vi "AssertsSubpanelExecStateIdleorRun.vi"(0 "VI Reference In":refnum<vi>, 1 "Label (VI Title)":string="Default", 11 "error in":errorcluster) -> (4 "VI Reference Out":refnum<vi>, 15 "error out":errorcluster)   [LabVIEW 2016, in "DronaTest.lvlib"]
uses:
  APIs/Stimulus/ControlValue/ValueSignalByPathString.vi
  APIs/Stimulus/ControlValue/ValueSignalLatchBooleanString.vi
  APIs/Assert/AssertSubpanel/AssertSubpanelVIExecIdle.vi
  <vilib>/addons/_JKI Toolkits/Caraya/classes/Assert/Assert Not Error.vi
  APIs/Assert/AssertSubpanel/AssertSubpanelVIExecRunning.vi
  APIs/Assert/AssertSubpanel/AssertSubpanelVIExecNotBad.vi
  DronaTest.lvlib
  <vilib>/addons/_JKI Toolkits/Caraya/classes/Test/Test.lvclass
  Drona.lvlib
  <vilib>/addons/_JKI Toolkits/Caraya/classes/Assert/Assert.lvclass
  APIs/Stimulus/ControlValue/ControlValue.lvlib
  APIs/Assert/AssertSubpanel/AssertSubpanel.lvlib
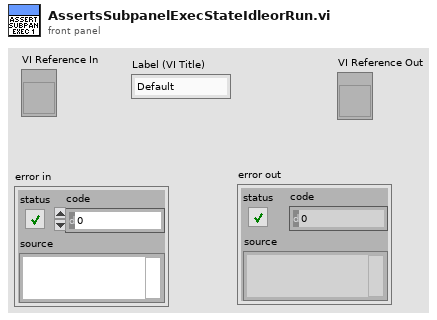
[diagram p1: front panel]
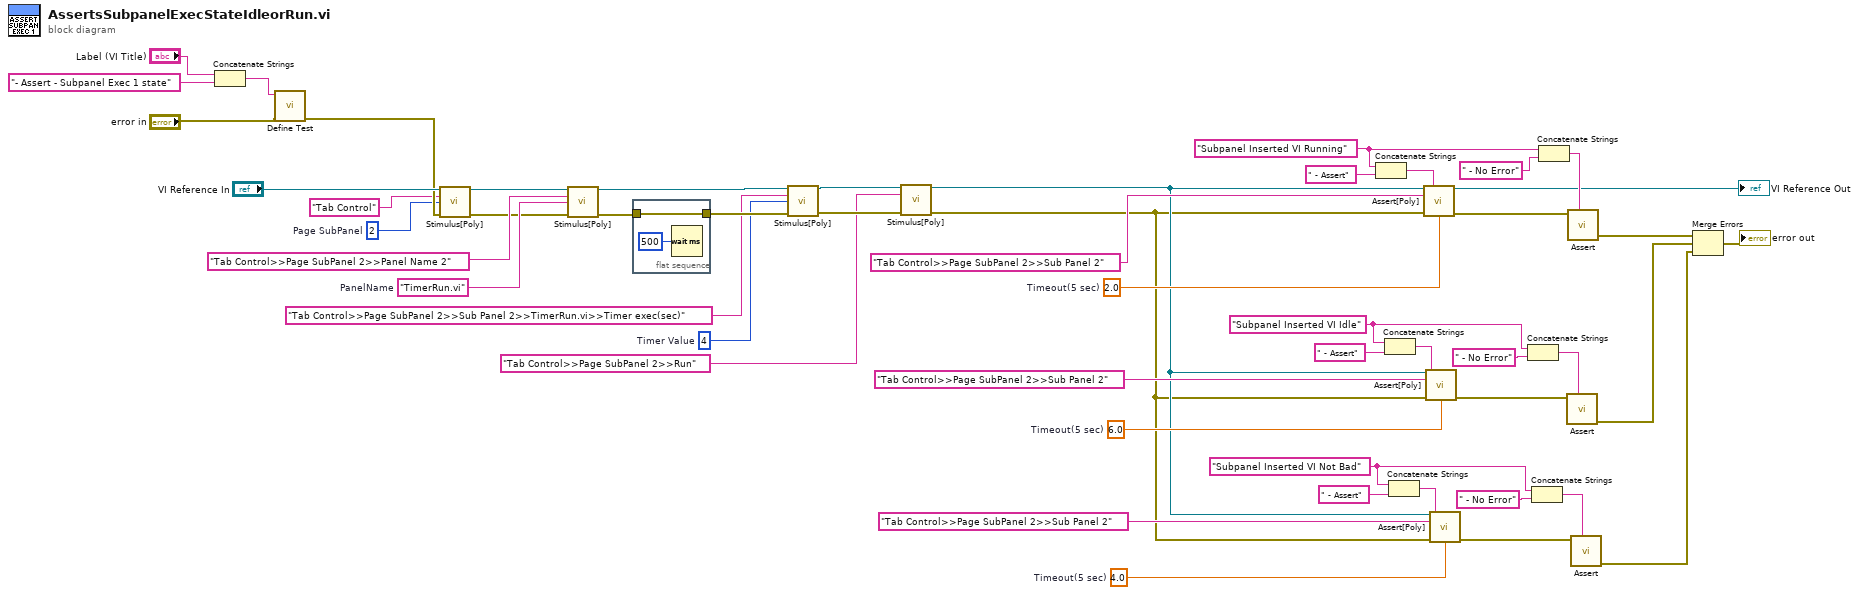
[diagram p0: block diagram]
diagram:
  w1 = 4.0  # Timeout(5 sec)
  w8 = "Subpanel Inserted VI Not Bad" ("Label")
  w16 = 4  # Timer Value
  w20 = 2  # Page SubPanel
  w26 = "TimerRun.vi"  # PanelName
  w36 = "Subpanel Inserted VI Idle" ("Label")
  w39 = "Subpanel Inserted VI Running" ("Label")
  w33 = 6.0  # Timeout(5 sec)
  w29 = 2.0  # Timeout(5 sec)
  n1 = Concatenate Strings("Label (VI Title)", "- Assert - Subpanel Exec 1 state" ("string")) -> (w46:string)
  n2 = call <vilib>:"Define Test.vi"("error in (no error)"="error in", "Label (VI Title)"=w46) -> ("error out"=w22:errorcluster)  [unwired: 9 in]
  n3 = call-poly "Stimulus[Poly].vi"("VI Reference In"="VI Reference In", "Control Path"="Tab Control", "Value (Signaling)"=w20, "error in"=w22) -> ("VI Reference Out"=w23:refnum<vi>, "error out"=w19:errorcluster)  [unwired: 10 in]
  n4 = call-poly "Stimulus[Poly].vi"("VI Reference In"=w23, "Control Path"="Tab Control>>Page SubPanel 2>>Panel Name 2", "Value (Signaling)"=w26, "error in"=w19) -> ("VI Reference Out"=w12:refnum<vi>, "error out"=w25:errorcluster)  [unwired: 10 in]
  n5 = flat-sequence {
    tunnel: w25 -> [w53]
    tunnel: [w53] -> w18
    frame #0 {
      n6 = Wait (ms)(milliseconds to wait=u32 500) -> ()  [unwired: 1 out]
    }
  }
  n7 = call-poly "Stimulus[Poly].vi"("VI Reference In"=w12, "Control Path"="Tab Control>>Page SubPanel 2>>Sub Panel 2>>TimerRun.vi>>Timer exec(sec)", "Value (Signaling)"=w16, "error in"=w18) -> ("VI Reference Out"=w15:refnum<vi>, "error out"=w14:errorcluster)  [unwired: 10 in]
  n8 = call-poly "Stimulus[Poly].vi"("VI Reference In"=w15, "Control Path"="Tab Control>>Page SubPanel 2>>Run", "error in"=w14) -> ("VI Reference Out"=w4:refnum<vi>, "error out"=w3:errorcluster)  [unwired: 11 in]
  n9 = Concatenate Strings(w39, " - Assert" ("string")) -> (w31:string)
  n10 = Concatenate Strings(w36, " - Assert" ("string")) -> (w35:string)
  n11 = Concatenate Strings(w8, " - Assert" ("string")) -> (w9:string)
  n12 = call-poly "Assert[Poly].vi"("VI Reference In"=w4, "Test Label"=w31, "Control Path"="Tab Control>>Page SubPanel 2>>Sub Panel 2", "Error In"=w3, "Timeout(5 sec)"=w29) -> ("VI Reference Out"=→"VI Reference Out":refnum<vi>, "Error Out"=w27:errorcluster)  [unwired: 9 in]
  n13 = call-poly "Assert[Poly].vi"("VI Reference In"=w4, "Test Label"=w35, "Control Path"="Tab Control>>Page SubPanel 2>>Sub Panel 2", "Error In"=w3, "Timeout(5 sec)"=w33) -> ("Error Out"=w32:errorcluster)  [unwired: 9 in, 1 out]
  n14 = call-poly "Assert[Poly].vi"("VI Reference In"=w4, "Test Label"=w9, "Control Path"="Tab Control>>Page SubPanel 2>>Sub Panel 2", "Error In"=w3, "Timeout(5 sec)"=w1) -> ("Error Out"=w11:errorcluster)  [unwired: 9 in, 1 out]
  n15 = Concatenate Strings(w36, " - No Error" ("string")) -> (w41:string)
  n16 = Concatenate Strings(w8, " - No Error" ("string")) -> (w6:string)
  n17 = Concatenate Strings(w39, " - No Error" ("string")) -> (w51:string)
  n18 = call-poly <vilib>:"Assert.vi"("Label"=w41, "Not Error?"=w32) -> ("error out"=w48:errorcluster)  [unwired: 9 in]
  n19 = call-poly <vilib>:"Assert.vi"("Label"=w51, "Not Error?"=w27) -> ("error out"=w49:errorcluster)  [unwired: 9 in]
  n20 = call-poly <vilib>:"Assert.vi"("Label"=w6, "Not Error?"=w11) -> ("error out"=w2:errorcluster)  [unwired: 9 in]
  n21 = Merge Errors(w49, w48, w2) -> (→"error out":errorcluster)
